vi "SV Limit Testing for Monitoring (waveform).vi"(7 "reset":bool, 9 "lower limit":dbl=-inf format="%.2f", 10 "upper limit":dbl=inf format="%.2f", 11 "signal in":waveform(dbl)) -> (1 "lower limit clearance":dbl=nan format="%.6f", 2 "upper limit clearance":dbl=nan format="%.6f", 3 "test passed?":bool, 5 "timestamp":timestamp format="%<%.6X\n%x>T")   [LabVIEW 2017]
doc: "Performs limit testing on waveforms, spectra, XY data, identified peaks, or scalar measurements. You can wire <B>output values</B> to a graph to view the limits, signal, and failures. Wire data to the<B> signal in</B> input to determine the polymorphic instance to use or manually select the instance."
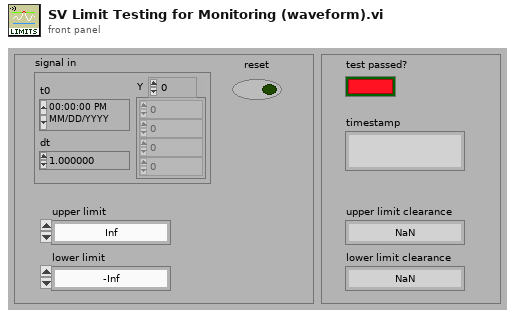
[diagram p1: front panel]
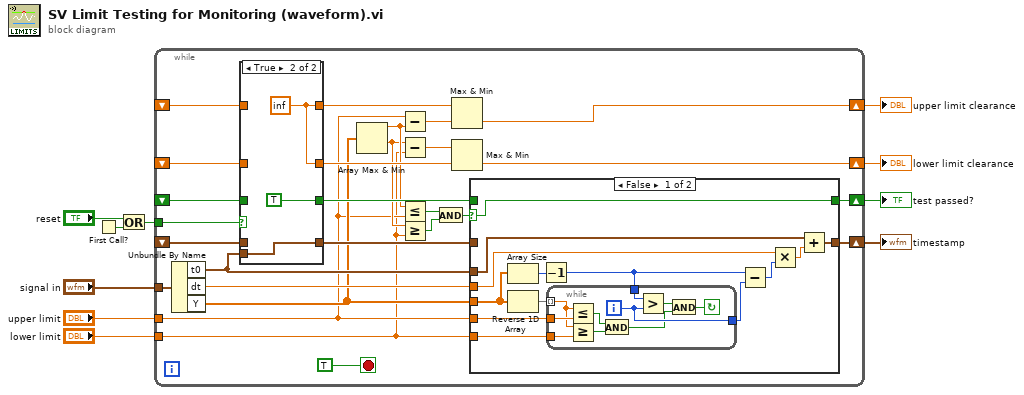
[diagram p0: block diagram]
diagram:
  n1 = First Call?() -> (First Call?: T/F=w2:bool)
  n2 = Or(x="reset", y=w2) -> (x .or. y?=w3:bool)
  n3 = while {
    tunnel: "signal in" -> [w37]
    tunnel: "upper limit" -> [w12]
    tunnel: "lower limit" -> [w11]
    shift-right: [w36] -> w7
    shift-left: _ -> [w33]
    shift-right: [w35] -> w6
    shift-left: _ -> [w31]
    shift-right: [w19] -> w5
    shift-left: _ -> [w29]
    shift-right: [w26] -> w1
    shift-left: _ -> [w28]
    tunnel: w3 -> [w34]
    stop <- TRUE stop-if-true
    n4 = Unbundle By Name(w37) -> ("t0"=w25:timestamp, "dt"=w24:dbl, "Y"=w13:dbl[])
    n5 = case shown="True" w34 {
      tunnel: w33 -> [w66 _]
      tunnel: [w66 w67] -> w32
      tunnel: w31 -> [w65 _]
      tunnel: [w65 w67] -> w30
      tunnel: w29 -> [w64 _]
      tunnel: [w64 TRUE] -> w20
      tunnel: w28 -> [w63 _]
      tunnel: [w63 w69] -> w27
      tunnel: w25 -> [_ w69]
      frame False {
      }
      frame True {
        w67 = inf
      }
    }
    n6 = Array Max & Min(array=w13) -> (max value=w16:dbl, min value=w15:dbl)  [unwired: 2 out]
    n7 = Subtract(x=w12, y=w16) -> (x-y=w18:dbl)
    n8 = Subtract(x=w15, y=w11) -> (x-y=w17:dbl)
    n9 = Less Or Equal?(x=w16, y=w12) -> (x <= y?=w22:bool)
    n10 = Greater Or Equal?(x=w15, y=w11) -> (x >= y?=w21:bool)
    n11 = And(x=w22, y=w21) -> (x .and. y?=w14:bool)
    n12 = Max & Min(x=w32, y=w18) -> (min(x,y)=w36:dbl)  [unwired: 1 out]
    n13 = Max & Min(x=w17, y=w30) -> (min(x,y)=w35:dbl)  [unwired: 1 out]
    n14 = case shown="False" w14 {
      selector: w14 -> [w47 _]
      tunnel: w27 -> [_ w62]
      tunnel: [w49 w62] -> w26
      tunnel: w25 -> [w50 _]
      tunnel: w24 -> [w46 _]
      tunnel: w20 -> [_ w61]
      tunnel: [w47 w61] -> w19
      tunnel: w13 -> [w38 _]
      tunnel: w12 -> [w45 _]
      tunnel: w11 -> [w44 _]
      frame False {
        n15 = Array Size(array=w38) -> (size(s)=w42:i32)
        n16 = Reverse 1D Array(array=w38) -> (reversed array=w43:dbl[])
        n17 = Decrement(x=w42) -> (x-1=w41:i32)
        n18 = while {
          tunnel: [w54] -> w40
          tunnel: w45 -> [w58]
          tunnel: w44 -> [w57]
          tunnel: w43 -> [w56] mode=indexing
          tunnel: w41 -> [w55]
          i -> [w54]
          stop <- w51 continue-if-true
          n19 = Less Or Equal?(x=w56, y=w58) -> (x <= y?=w60:bool)
          n20 = Greater Or Equal?(x=w56, y=w57) -> (x >= y?=w59:bool)
          n21 = And(x=w60, y=w59) -> (x .and. y?=w52:bool)
          n22 = Greater?(x=w55, y=w54) -> (0:w53:bool)
          n23 = And(x=w53, y=w52) -> (x .and. y?=w51:bool)
        }
        n24 = Subtract(x=w41, y=w40) -> (x-y=w39:i32)
        n25 = Multiply(x=w46, y=w39) -> (x*y=w48:dbl)
        n26 = Add(x=w50, y=w48) -> (x+y=w49:timestamp)
      }
      frame True {
      }
    }
  }
  "test passed?" <- w5
  "upper limit clearance" <- w7
  "lower limit clearance" <- w6
  "timestamp" <- w1
